vi "Save-Close Word Report.vi"(7 "File Path":string, 8 "error in (no error)":errorcluster, 9 "Certificate File Name":string, 10 "Base Folder Path":string="C:\\Teststand\\Certificates", 11 "report in":refnum<class "NI_report.lvclass">) -> (0 "error out":errorcluster)   [LabVIEW 2014]
uses:
  <vilib>/Utility/NIReport.llb/NI_report.lvclass
  CustomControls/TSE_Status.ctl
  CustomControls/Program_States.ctl
  <vilib>/Utility/NIReport.llb/Word/NI_Word.lvclass
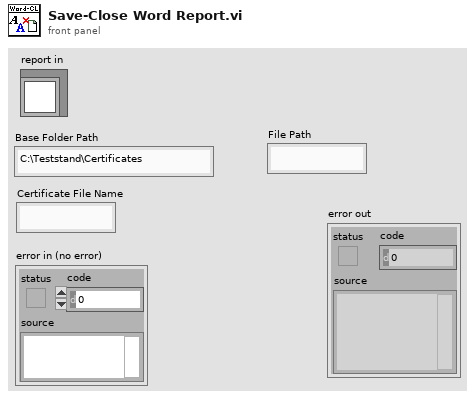
[diagram p1: front panel]
types:
  T1 = typedef "TSE_Status.ctl" = cluster{"Return Code":i32, "Message":string, "error in (no error)":errorcluster, "Program State":T2, "Test A. Suresi":u32}
  T2 = typedef "Program_States.ctl" = enum16{"Ön Yükleme", "TSE Baslat", "Kalibratöre Baglan", "Kalibratörü Baslat", "Ön Yükleme Tamam", "Frekans Testi", "Gerilim Testi", "Akim Testi", "Aktif Guc Testi", "Reaktif Guc Testi", "AC Akim Harmonik Testi", "AC Gerilim Harmonik Testi", "Flicker Testi", "Rapor Cikarma", "Yeniden Başlat", "Bekleme", "Durdur"}
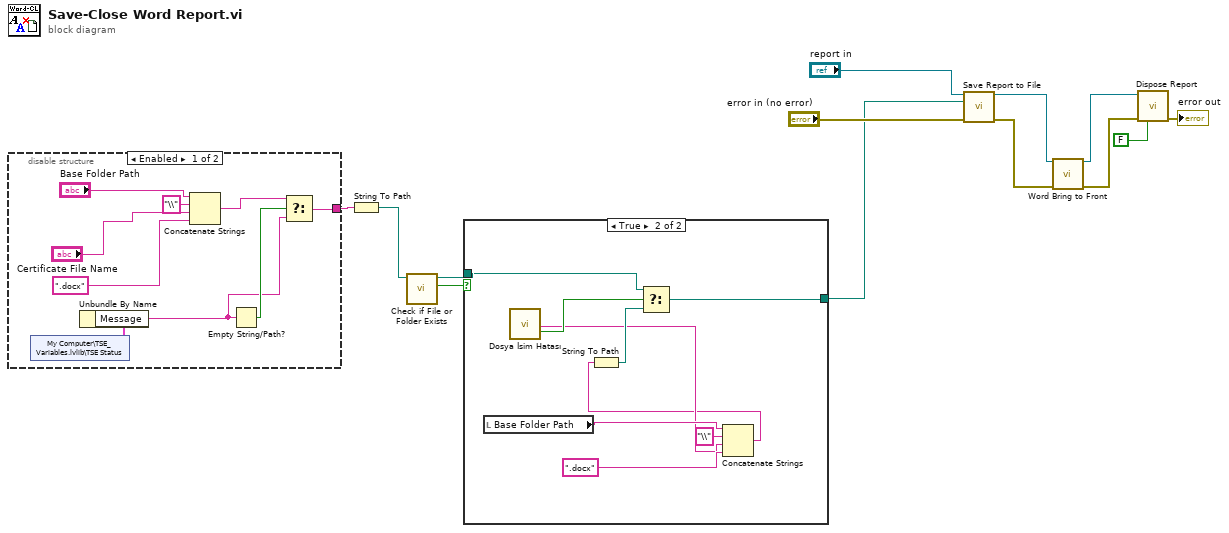
[diagram p0: block diagram]
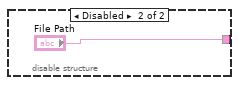
[diagram p3: hidden frame]
diagram:
  n1 = disable-structure shown="Enabled" {
    disable-tunnel: [w17 "File Path"] -> w10
    frame Enabled {
      n2 = shared-variable "My Computer\\TSE_Variables.lvlib\\TSE Status"() -> (w18:T1)  [unwired: 1 in, 1 out]
      n3 = Unbundle By Name(w18) -> ("Message"=w14:string)
      n4 = Concatenate Strings("Base Folder Path", "\\" ("string"), "Certificate File Name", ".docx" ("string")) -> (w15:string)
      n5 = Empty String/Path?(string/path=w14) -> (empty?=w16:bool)
      n6 = Select(t=w15, s=w16, f=w14) -> (s? t:f=w17:string)
    }
    frame Disabled {
    }
  }
  n7 = String To Path(string=w10) -> (path=w4:path)
  n8 = call <vilib>:"Check if File or Folder Exists.vi"("path"=w4) -> ("file or folder exists?"=w3:bool, "dup path"=w2:path)  [unwired: 8 in, 1 out]
  n9 = case shown="True" w3 {
    tunnel: w2 -> [w24 w32]
    tunnel: [w24 w31] -> w1
    frame False {
    }
    frame True {
      n10 = local read "Base Folder Path"() -> (w29:string)
      n11 = call "Dosya İsim Hatası"() -> ("Yeni Dosya İsmi"=w26:string, "Üzerine Yaz"=w33:bool)  [unwired: 17 in, 1 out]
      n12 = Concatenate Strings(w29, "\\" ("string"), w26, ".docx" ("string")) -> (w25:string)
      n13 = String To Path(string=w25) -> (path=w30:path)
      n14 = Select(t=w32, s=w33, f=w30) -> (s? t:f=w31:path)
    }
  }
  n15 = call-dynamic "Save Report to File.vi"("report in"="report in", "report file path"=w1, "error in (no error)"="error in (no error)") -> ("report out"=w8:refnum<class "NI_report.lvclass">, "error out"=w6:errorcluster)  [unwired: 11 in]
  n16 = call <vilib>:"Word Bring to Front.vi"("report in"=w8, "error in (no error)"=w6) -> ("report out"=w7:refnum<class "NI_report.lvclass">, "error out"=w5:errorcluster)  [unwired: 12 in]
  n17 = call-dynamic "Dispose Report.vi"("report in"=w7, "error in (no error)"=w5, "close report? (T)"=FALSE ("Close Report? (T)")) -> ("error out"=→"error out":errorcluster)  [unwired: 12 in]
